vi "SD-Wait (ms)__ogtk.vi"(8 "error in (no error)":errorcluster, 9 "Abort wait on occurence":refnum<k4>, 10 "Wait on Error (FALSE)":bool, 11 "milliseconds to wait":u32) -> (0 "error out":errorcluster, 3 "millisecond timer value":u32)   [LabVIEW 2020, in "SD-openg_time.lvlib"]
doc: "Wait (ms) primitive with added error handling. This VI will not wait if an error is passed into it unless the <B>Wait on Error</B> input is set to TRUE."
uses:
  SD-openg_time.lvlib
panel:
  # "[OpenG VI Tags] ***Do Not Remove***"
  # "Wait (ms).vi\n\nWait (ms) primitive with added error handling\n\nPlease visit http://www.OpenG.org to learn about the\nOpen Source LabVIEW software movement.\n\nNOTICE -- YOU MUST LEAVE THIS NOTICE IN PLACE.  PER THE TERMS OF THE LICENSE BELOW, YOU MAY SUBLICENSE THIS SOFTWARE \nIN ANY WAY THAT DOES NOT CONFLICT WITH THIS LICENSE.\n\n### BSD License (http://www.opensource.org/licenses/bsd-license.php) Begin ###\n \nCopyright (c) 2002, Jean-Pierre Drolet <drolet_jp@hotmail.com>\nCopyright (c) 2002, Jim Kring <jim@jimkring.com>\n\nAll rights reserved.\n\nRedistribution and use in source and binary forms, with or without modification, are permitted provided that the following conditions are met:\n\n    * Redistributions of source code must retain the above copyright notice, this list of conditions and the following disclaimer.\n    * Redistributions in binary form must reproduce the above copyright notice, this list of conditions and the following disclaimer in the \n       documentation and/or other materials provided with the distribution.\n    * Neither the name of SciWare, James Kring, Inc., nor the names of its contributors may be used to endorse or promote products derived \n       from this software without specific prior written permission.\n\nTHIS SOFTWARE IS PROVIDED BY THE COPYRIGHT HOLDERS AND CONTRIBUTORS \"AS IS\" AND ANY EXPRESS OR IMPLIED WARRANTIES, \nINCLUDING, BUT NOT LIMITED TO, THE IMPLIED WARRANTIES OF MERCHANTABILITY AND FITNESS FOR A PARTICULAR PURPOSE ARE \nDISCLAIMED. IN NO EVENT SHALL THE COPYRIGHT OWNER OR CONTRIBUTORS BE LIABLE FOR ANY DIRECT, INDIRECT, INCIDENTAL,\n SPECIAL, EXEMPLARY, OR CONSEQUENTIAL DAMAGES (INCLUDING, BUT NOT LIMITED TO, PROCUREMENT OF SUBSTITUTE GOODS OR \nSERVICES; LOSS OF USE, DATA, OR PROFITS; OR BUSINESS INTERRUPTION) HOWEVER CAUSED AND ON ANY THEORY OF LIABILITY, \nWHETHER IN CONTRACT, STRICT LIABILITY, OR TORT (INCLUDING NEGLIGENCE OR OTHERWISE) ARISING IN ANY WAY OUT OF THE USE \nOF THIS SOFTWARE, EVEN IF ADVISED OF THE POSSIBILITY OF SUCH DAMAGE.\n\n### BSD License End ###"
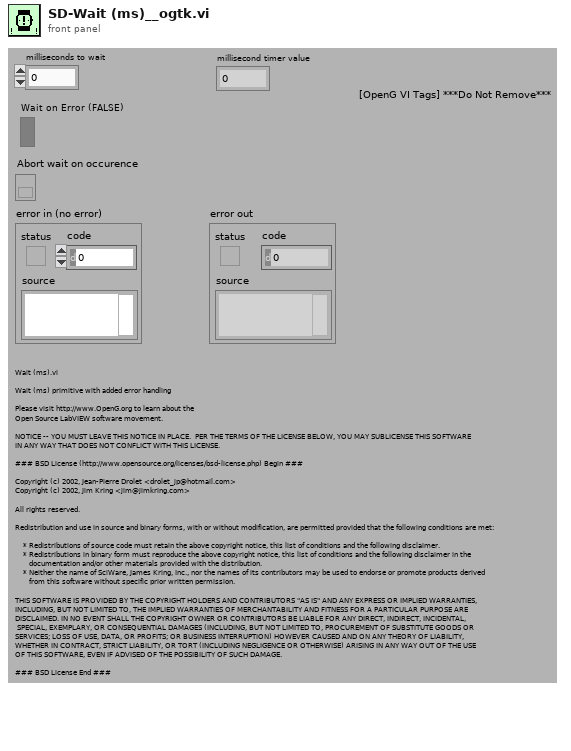
[diagram p1: front panel]
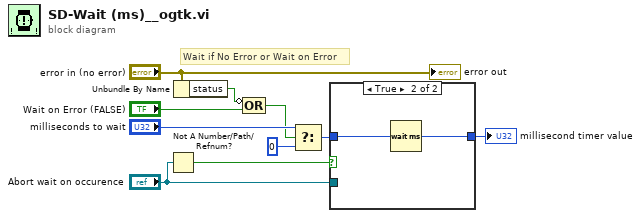
[diagram p0: block diagram]
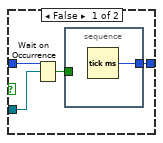
[diagram p2: hidden frame]
diagram:
  # "Wait if No Error or Wait on Error"
  n1 = Not A Number/Path/Refnum?(number/path/refnum="Abort wait on occurence") -> (NaN/Path/Refnum?=w2:bool)
  n2 = Unbundle By Name("error in (no error)") -> ("status"=w8:bool)
  n3 = Compound Arithmetic op=OR(invert w8, "Wait on Error (FALSE)") -> (w6:bool)
  n4 = Select(t="milliseconds to wait", s=w6, f=u32 0) -> (s? t:f=w5:u32)
  n5 = case shown="True" w2 {
    tunnel: w5 -> [w14 w17]
    tunnel: [w11 w16] -> w3
    tunnel: "Abort wait on occurence" -> [w13 _]
    frame False {
      n6 = Wait on Occurrence(2:w13, 3:w14) -> (0:w12:bool)  [unwired: 1 in]
      n7 = stacked-sequence {
        tunnel: w12 -> [_]
        tunnel: [w15] -> w11
        frame #0 {
          n8 = Tick Count (ms)() -> (millisecond timer value=w15:u32)
        }
      }
    }
    frame True {
      n9 = Wait (ms)(milliseconds to wait=w17) -> (millisecond timer value=w16:u32)
    }
  }
  "millisecond timer value" <- w3
  "error out" <- "error in (no error)"
